vi "BuscaAmplitudePolo.vi"(1 "Config":T1={"Componentes"=[{"Pólo:"=0, "Amplitude:"=0.0}, {"Pólo:"=0, "Amplitude:"=0.0}, {"Pólo:"=0, "Amplitude:"=0.0}, {"Pólo:"=0, "Amplitude:"=0.0}], "Num Polos"=0, "Folga Nominal"=0.0, "Ruido"=0.0, "Saturacao"=0.0, "Angulo"=0.0}, 4 "polo":u16) -> (16 "Amp. Polo":dbl)   [LabVIEW 2017]
uses:
  Typedefs/Tipo_ParamsEntreferro.ctl
  Typedefs/Tipo_ComponenteSinalEntreferro.ctl
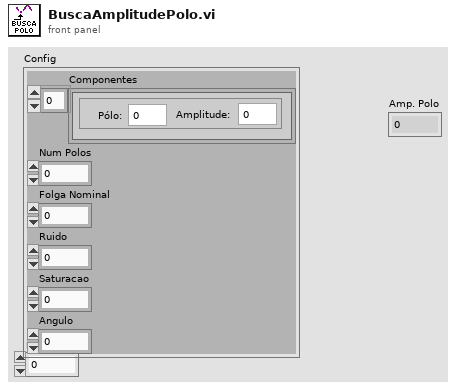
[diagram p1: front panel]
types:
  T1 = typedef "Tipo_ParamsEntreferro.ctl" = cluster{"Componentes":T2[], "Num Polos":u16, "Folga Nominal":dbl, "Ruido":dbl, "Saturacao":dbl, "Angulo":dbl}
  T2 = typedef "Tipo_ComponenteSinalEntreferro.ctl" = cluster{"Pólo:":u16, "Amplitude:":dbl}
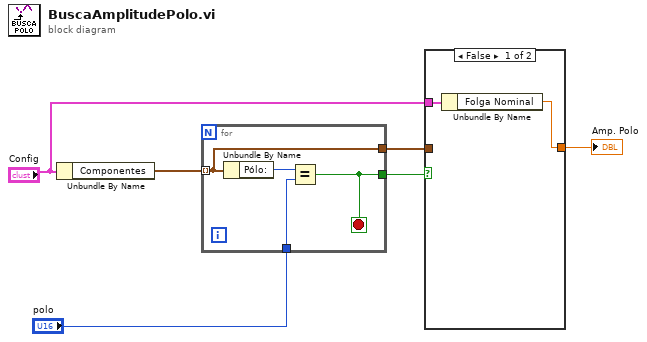
[diagram p0: block diagram]
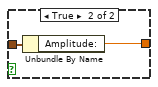
[diagram p2: hidden frame]
diagram:
  n1 = Unbundle By Name("Config") -> ("Componentes"=w6:T2[])
  n2 = for {
    tunnel: w6 -> [w7] mode=indexing
    tunnel: "polo" -> [w9]
    tunnel: [w8] -> w4
    tunnel: [w7] -> w3
    stop <- w8 stop-if-true
    n3 = Unbundle By Name(w7) -> ("Pólo:"=w10:u16)
    n4 = Equal?(x=w10, y=w9) -> (x = y?=w8:bool)
  }
  n5 = case shown="False" w4 {
    tunnel: w3 -> [_ w14]
    tunnel: [w11 w13] -> w2
    tunnel: "Config" -> [w12 _]
    frame False {
      n6 = Unbundle By Name(w12) -> ("Folga Nominal"=w11:dbl)
    }
    frame True {
      n7 = Unbundle By Name(w14) -> ("Amplitude:"=w13:dbl)
    }
  }
  "Amp. Polo" <- w2
